vi "NXT_ Init Message Data.vi"() -> (0 "_messageData":T1)   [LabVIEW 2012, in "Tugboat.lvrbt"]
uses:
  Tugboat.lvrbt
  messageData_t.ctl
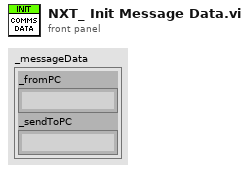
[diagram p1: front panel]
types:
  T1 = typedef "messageData_t.ctl" = cluster{"_fromPC":string, "_sendToPC":string}
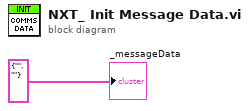
[diagram p0: block diagram]
diagram:
  "_messageData" <- T1 {"_fromPC"="", "_sendToPC"=""} ("_messageData")
